vi "AcquireImage.vi"(8 "error in (no error)":errorcluster, 11 "Photometrics Cam v2 in":refnum<class "Photometrics_CH-250_Cam.lvclass">) -> (0 "error out":errorcluster, 1 "OK":bool, 3 "Photometrics Cam v2 out":refnum<class "Photometrics_CH-250_Cam.lvclass">)   [LabVIEW 2013, in "Photometrics_CH-250_Cam.lvclass"]
uses:
  Photometrics_CH-250_Cam.lvclass
  CameraSessionClass/CS250-CameraHardwareClass.lvclass
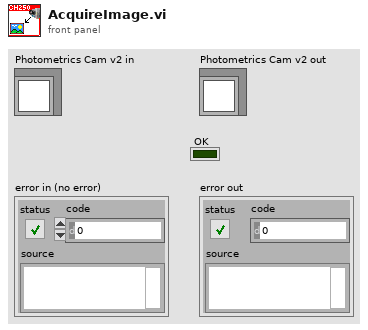
[diagram p1: front panel]
types:
  T1 = typedef "IMAQ Image.ctl" = refnum<image>
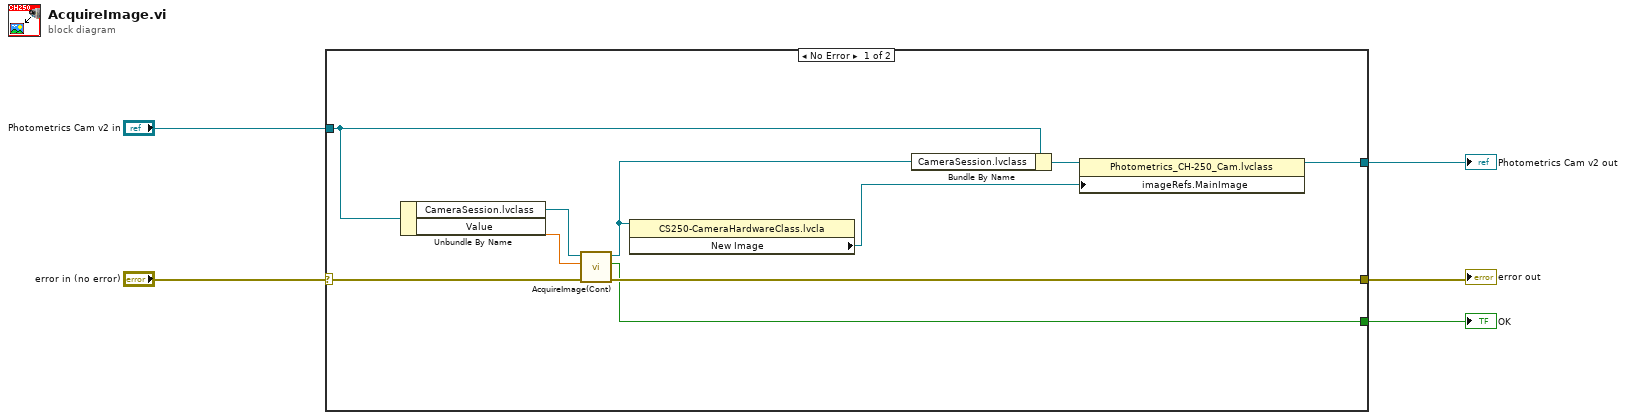
[diagram p0: block diagram]
diagram:
  n1 = case shown="No Error" "error in (no error)" {
    selector: "error in (no error)" -> [w11 w17]
    tunnel: "Photometrics Cam v2 in" -> [w9 w16]
    tunnel: [w15 w17] -> w4
    tunnel: [w7 w16] -> w3
    tunnel: [w12 _] -> w2
    frame No Error {
      n2 = Unbundle By Name(w9) -> ("CameraSession.lvclass"=w13:refnum<class "CS250-CameraHardwareClass.lvclass">, "Value"=w14:dbl)
      n3 = call-dynamic "AcquireImage(Cont).vi"("error in (no error)"=w11, "timeout (s)"=w14, "CameraSession in"=w13) -> ("error out"=w15:errorcluster, "ready"=w12:bool, "CameraSession out"=w10:refnum<class "CS250-CameraHardwareClass.lvclass">)  [unwired: 6 in]
      n4 = property class="CS250-CameraHardwareClass.lvcla"(reference=w10) -> ("New Image"=w6:T1)  [unwired: 1 in, 2 out]
      n5 = Bundle By Name(cluster=w9, "CameraSession.lvclass"=w10) -> (w8:refnum<class "Photometrics_CH-250_Cam.lvclass">)
      n6 = property class="Photometrics_CH-250_Cam.lvclass"(reference=w8, "imageRefs.MainImage"=w6) -> (reference out=w7:refnum<class "Photometrics_CH-250_Cam.lvclass">)  [unwired: 1 in, 1 out]
    }
    frame Error {
    }
  }
  "error out" <- w4
  "Photometrics Cam v2 out" <- w3
  "OK" <- w2
